vi "ComputerName.vi"(2 "error in (no error)":errorcluster) -> (0 "error out":errorcluster, 1 "String/Binary data":string)   [LabVIEW 2021]
uses:
  <vilib>/registry/registry.llb/Registry RtKey.ctl
  <vilib>/registry/registry.llb/Registry SAM.ctl
  <vilib>/registry/registry.llb/Read Registry Value Simple STR.vi
panel:
  in  "value":string="ComputerName"
  in  "root key (HKEY_LOCAL_MACHINE)":T1=enum."HKEY_LOCAL_MACHINE"
  in  "subkey":string="System\\CurrentControlSet\\Control\\ComputerName\\ComputerName"
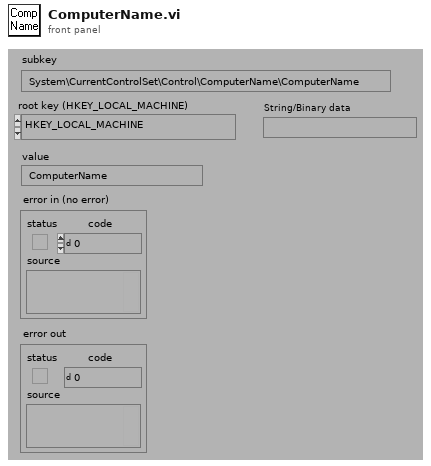
[diagram p1: front panel]
types:
  T1 = typedef "Registry RtKey.ctl" = enum32{"HKEY_CLASSES_ROOT", "HKEY_CURRENT_USER", "HKEY_LOCAL_MACHINE", "HKEY_USERS", "HKEY_PERFORMANCE_DATA", "HKEY_CURRENT_CONFIG", "HKEY_DYN_DATA"}
  T2 = typedef "Registry SAM.ctl" = enum32{"KEY_QUERY_VALUE", "KEY_SET_VALUE", "KEY_CREATE_SUB_KEY", "KEY_ENUMERATE_SUB_KEYS", "KEY_NOTIFY", "KEY_CREATE_LINK", "KEY_READ", "KEY_WRITE", "KEY_ALL_ACCESS", "KEY_READ | KEY_WRITE"}
  T3 = typedef "Registry refnum.ctl" = refnum<k1>
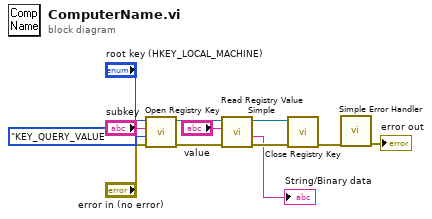
[diagram p0: block diagram]
diagram:
  n1 = call <vilib>:"Open Registry Key.vi"("error in (no error)"="error in (no error)", "security access mask (KEY_READ | KEY_WRITE)"=Registry_SAM."KEY_QUERY_VALUE", "subkey"="subkey", "root key (HKEY_LOCAL_MACHINE)"="root key (HKEY_LOCAL_MACHINE)") -> ("error out"=w12:errorcluster, "refnum out"=w11:T3)  [unwired: 6 in]
  n2 = call-poly <vilib>:"Read Registry Value Simple.vi"("error in (no error)"=w12, "value"="value", "refnum"=w11) -> ("error out"=w10:errorcluster, "String/Binary data"=→"String/Binary data":string, "refnum out"=w9:T3)  [unwired: 3 in, 1 out]
  n3 = call <vilib>:"Close Registry Key.vi"("error in (no error)"=w10, "refnum"=w9) -> ("error out"=w8:errorcluster)  [unwired: 5 in]
  n4 = call <vilib>:"Simple Error Handler.vi"("error in (no error)"=w8) -> ("error out"=→"error out":errorcluster)  [unwired: 4 in, 4 out]
